vi "came_from.vi"(10 "Node":cluster{"Weight":dbl, "Row":dbl, "Col":dbl}, 11 "Came_from":T1(array[cluster])) -> (3 "Node came from":cluster{"Weight":dbl, "Row":dbl, "Col":dbl})   [LabVIEW 2014]
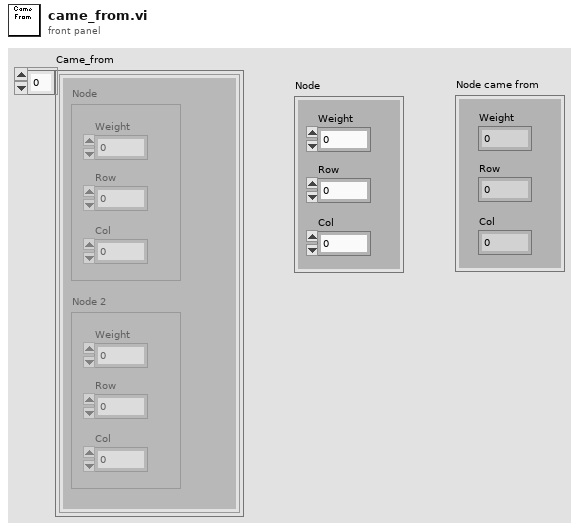
[diagram p1: front panel]
types:
  T1 = cluster{"Node":cluster{"Weight":dbl, "Row":dbl, "Col":dbl}, "Node 2":cluster{"Weight":dbl, "Row":dbl, "Col":dbl}}[]
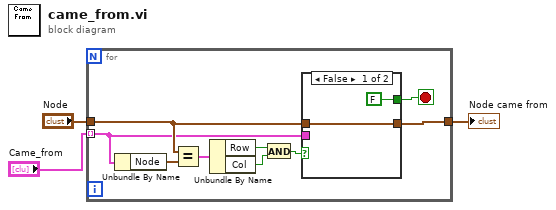
[diagram p0: block diagram]
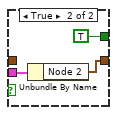
[diagram p2: hidden frame]
diagram:
  n1 = for {
    tunnel: "Came_from" -> [w10] mode=indexing
    tunnel: "Node" -> [w11]
    tunnel: [w9] -> w1
    stop <- w8 stop-if-true
    n2 = Unbundle By Name(w10) -> ("Node"=w12:cluster{"Weight":dbl, "Row":dbl, "Col":dbl})
    n3 = Equal?(x=w11, y=w12) -> (x = y?=w7:cluster{"Weight":bool, "Row":bool, "Col":bool})
    n4 = Unbundle By Name(w7) -> ("Row"=w6:bool, "Col"=w5:bool)
    n5 = And(x=w6, y=w5) -> (x .and. y?=w4:bool)
    n6 = case shown="False" w4 {
      tunnel: w11 -> [w14 _]
      tunnel: w10 -> [_ w17]
      tunnel: [w14 w16] -> w9
      tunnel: [FALSE TRUE] -> w8
      frame False {
      }
      frame True {
        n7 = Unbundle By Name(w17) -> ("Node 2"=w16:cluster{"Weight":dbl, "Row":dbl, "Col":dbl})
      }
    }
  }
  "Node came from" <- w1
